vi "NGTS_DAQmx_Eliminate Duplicate SCXI Tasks.vi"(7 "Tasknames In":string[](array[string]), 9 "Type of IO":enum16{"AI", "AO", "DI", "DO"}(ring)) -> (8 "Filtered Tasknames Out":string[](array[string]))   [LabVIEW 2018]
doc: "Takes in a list of PXI and SCXI modules used for the definition of DAQmx tasks, in the form PXInMody or SCxMody. Leaves all of the PXI modules as-is, as we want to create a task for each separate module. Filters the list of SCXI modules so that there is only a single task for each SCXI chassis; this is necessary for AI functions, as we must have only a single task for all AI functions for each chassis. Otherwise we get a sharing error. We also tag each SCXI task with its type (AI, AO, DI, DO) so that there are unique tasknames for each operation.\n\nBob Hamburger 2008-02-12"
uses:
  <userlib>/_OpenG.lib/array/array.llb/Remove Duplicates from 1D Array (String)__ogtk.vi
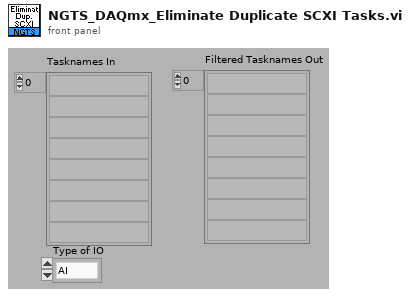
[diagram p1: front panel]
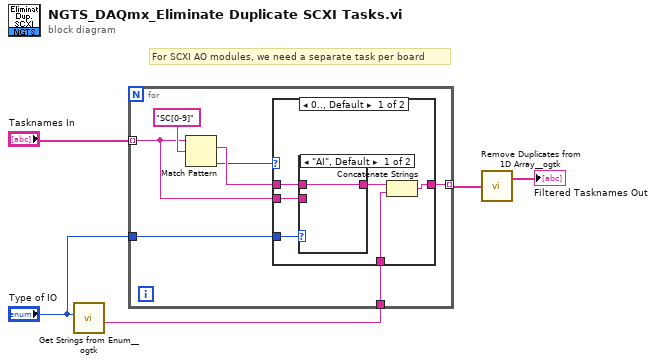
[diagram p0: block diagram]
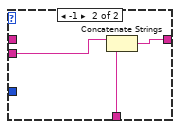
[diagram p3: hidden frame]
diagram:
  # "For SCXI AO modules, we need a separate task per board"
  n1 = call <userlib>:"Get Strings from Enum__ogtk.vi"("Enum"="Type of IO") -> ("String Value"=w3:string)  [unwired: 7 in, 3 out]
  n2 = for {
    tunnel: "Tasknames In" -> [w9] mode=indexing
    tunnel: [w10] -> w5 mode=indexing
    tunnel: w3 -> [w8]
    tunnel: "Type of IO" -> [w6]
    n3 = Match Pattern(string=w9, regular expression="SC[0-9]") -> (match substring=w11:string, offset past match=w7:i32)  [unwired: 1 in, 2 out]
    n4 = case shown="0.., Default" w7 {
      tunnel: [w18 w23] -> w10
      tunnel: w11 -> [w15 _]
      tunnel: w9 -> [w13 w21]
      tunnel: w8 -> [w17 w22]
      tunnel: w6 -> [w16 _]
      frame 0.., Default {
        n5 = case shown="\"AI\", Default" w16 {
          tunnel: [w19 w20] -> w14
          tunnel: w15 -> [w19 _]
          tunnel: w13 -> [_ w20]
          frame "AI", Default {
          }
          frame "AO" {
          }
        }
        n6 = Concatenate Strings(w14, w17) -> (w18:string)
      }
      frame -1 {
        n7 = Concatenate Strings(w21, w22) -> (w23:string)
      }
    }
  }
  n8 = call-poly <userlib>:"Remove Duplicates from 1D Array__ogtk.vi"("Input Array"=w5) -> ("Output Array"=→"Filtered Tasknames Out":string[])  [unwired: 1 out]
